vi "Record Minimum Distance.vi"(8 "Column":i32, 9 "Row":i32, 10 "Minimum Distance Matrix":u32[][](array[numeric]), 11 "Main Matrix":u8[][](array[numeric])) -> (0 "Columns Out":i32[](array[numeric]), 1 "Rows Out":i32[](array[numeric]), 2 "Minimum Distance Matrix Out":u32[][](array[numeric]))   [LabVIEW 2019, in "Day 15.lvlib"]
uses:
  Day 15.lvlib
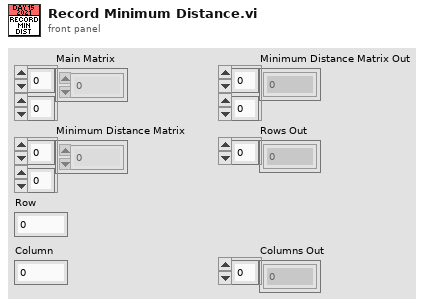
[diagram p1: front panel]
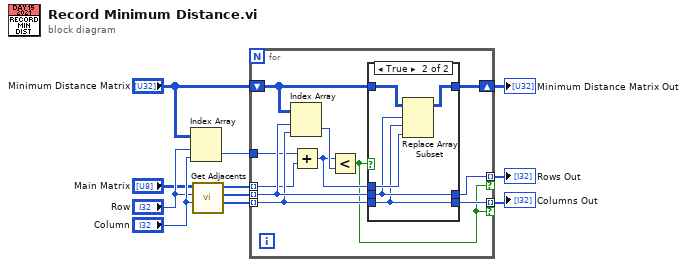
[diagram p0: block diagram]
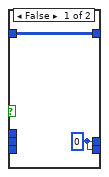
[diagram p2: hidden frame]
diagram:
  n1 = Index Array(array="Minimum Distance Matrix", index (row)="Row", index (col)="Column") -> (element=w11:u32)
  n2 = call "Get Adjacents.vi"("Column"="Column", "Row"="Row", "Array"="Main Matrix") -> ("Columns Out"=w7:i32[], "Rows Out"=w6:i32[], "Values"=w5:u8[])  [unwired: 6 in]
  n3 = for {
    tunnel: w5 -> [w16] mode=indexing
    tunnel: w6 -> [w20] mode=indexing
    tunnel: w7 -> [w19] mode=indexing
    shift-right: [w18] -> w3
    shift-left: "Minimum Distance Matrix" -> [w21]
    tunnel: w11 -> [w17]
    tunnel: [w14] -> w2 mode=indexing if=w12
    tunnel: [w13] -> w1 mode=indexing if=w12
    n4 = Index Array(array=w21, index (row)=w20, index (col)=w19) -> (element=w22:u32)
    n5 = Add(x=w17, y=w16) -> (x+y=w15:u32)
    n6 = Less?(x=w15, y=w22) -> (x < y?=w12:bool)
    n7 = case shown="True" w12 {
      tunnel: w21 -> [w24 w29]
      tunnel: w20 -> [_ w26]
      tunnel: w19 -> [_ w25]
      tunnel: w15 -> [_ w28]
      tunnel: [w24 w27] -> w18
      tunnel: [w23 w26] -> w14
      tunnel: [w23 w25] -> w13
      frame False {
        w23 = 0 ("Row Out")
      }
      frame True {
        n8 = Replace Array Subset(array=w29, new element=w28, index (row)=w26, index (col)=w25) -> (w27:u32[][])
      }
    }
  }
  "Minimum Distance Matrix Out" <- w3
  "Rows Out" <- w2
  "Columns Out" <- w1
